vi "Configure Analysis.vi"(0 "VISA resource name":refnum<visa-resource-name>, 1 "Range Coupling (F:Disable)":bool, 2 "Peak Excursion (3.0)":dbl=3.0 format="%^.2e", 3 "Peak Polarity (0: Positive)":u16(ring) items=["Positive", "Negative", "Both"], 4 "Partial Range Analysis State (F:Disable)":bool, 5 "error in (no error)":errorcluster, 6 "Channel (1)":i32=1, 7 "Target Value (0.0)":dbl format="%^.2e", 8 "Analysis Type (0: Peak to Peak)":u16(ring) items=["Peak to Peak", "Standard Deviation", "Mean", "Maximum", "Minimum", "Peak", "All Peaks", "All Targets"], 9 "Target Polarity (0: Positive)":u16(ring) items=["Positive", "Negative", "Both"], 10 "Start (0.0)":dbl format="%^.2e", 11 "Stop (0.0)":dbl format="%^.2e") -> (14 "VISA resource name out":refnum<visa-resource-name>, 19 "error out":errorcluster)   [LabVIEW 2022 SP3, in "Agilent ENA Series.lvlib"]
doc: "Configures the analysis parameters.\n\n<b>Note:</b>\nThis VI is not supported by the E5080A and E5080B."
uses:
  <instrlib>/Agilent ENA Series/Agilent ENA Series.lvlib
panel:
  # "Note:\nThis VI is not supported by the E5080A and E5080B."
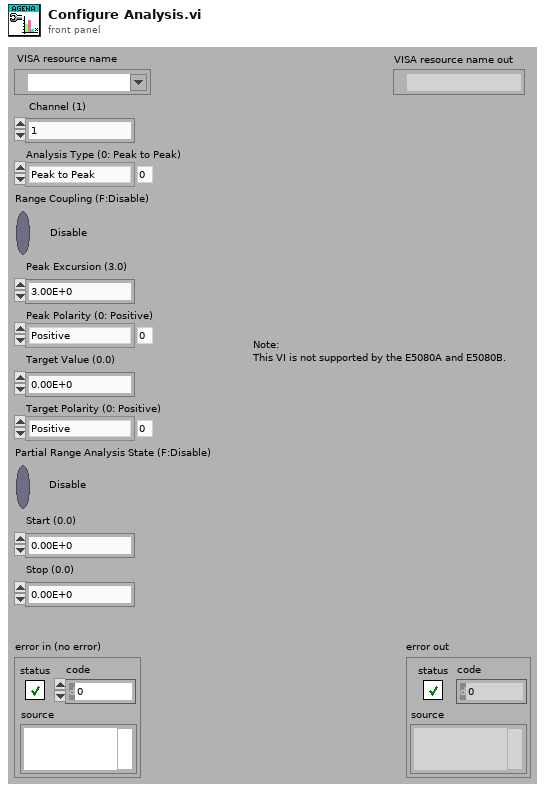
[diagram p1: front panel]
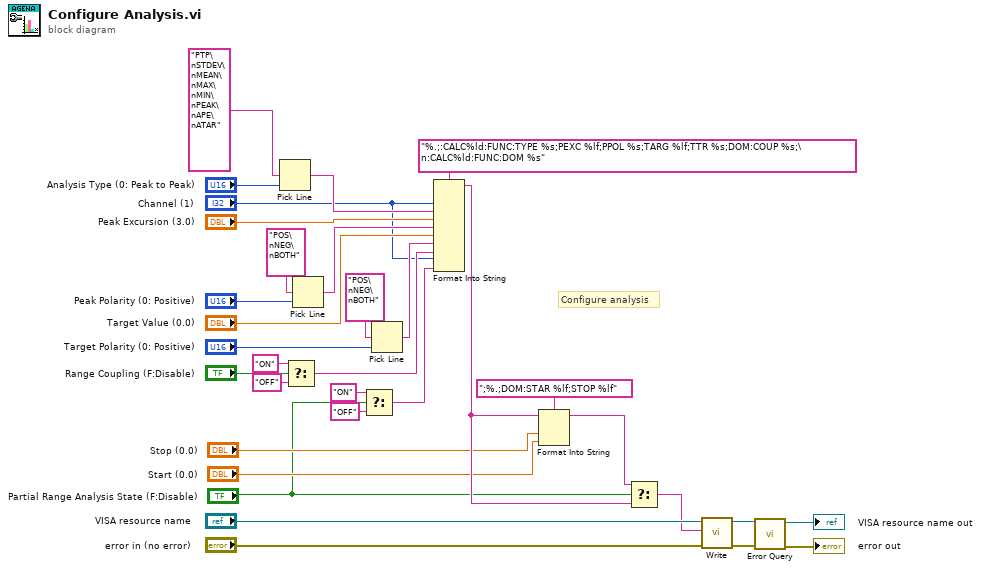
[diagram p0: block diagram]
diagram:
  # "Configure analysis"
  n1 = Pick Line(multi-line string="PTP\nSTDEV\nMEAN\nMAX\nMIN\nPEAK\nAPE\nATAR", line index="Analysis Type (0: Peak to Peak)") -> (output string=w25:string)  [unwired: 1 in]
  n2 = Select(t="ON", s="Range Coupling (F:Disable)", f="OFF") -> (s? t:f=w16:string)
  n3 = Pick Line(multi-line string="POS\nNEG\nBOTH", line index="Peak Polarity (0: Positive)") -> (output string=w21:string)  [unwired: 1 in]
  n4 = Select(t="ON", s="Partial Range Analysis State (F:Disable)", f="OFF") -> (s? t:f=w2:string)
  n5 = Pick Line(multi-line string="POS\nNEG\nBOTH", line index="Target Polarity (0: Positive)") -> (output string=w17:string)  [unwired: 1 in]
  n6 = Format Into String(format string="%.;:CALC%ld:FUNC:TYPE %s;PEXC %lf;PPOL %s;TARG %lf;TTR %s;DOM:COUP %s;\n:CALC%ld:FUNC:DOM %s", "Channel (1)", w25, "Peak Excursion (3.0)", w21, "Target Value (0.0)", w17, w16, "Channel (1)", w2) -> (resulting string=w10:string)  [unwired: 2 in, 1 out]
  n7 = Format Into String(format string=";%.;DOM:STAR %lf;STOP %lf", initial string=w10, "Stop (0.0)", "Start (0.0)") -> (resulting string=w9:string)  [unwired: 1 in, 1 out]
  n8 = Select(t=w9, s="Partial Range Analysis State (F:Disable)", f=w10) -> (s? t:f=w6:string)
  n9 = call <instrlib>:"Write.vi"("error in (no error)"="error in (no error)", "String ()"=w6, "VISA resource name"="VISA resource name") -> ("error out"=w14:errorcluster, "VISA resource name out"=w15:refnum<visa-resource-name>)  [unwired: 6 in, 1 out]
  n10 = call <instrlib>:"Error Query.vi"("error in (no error)"=w14, "VISA resource name"=w15) -> ("error out"=→"error out":errorcluster, "VISA resource name out"=→"VISA resource name out":refnum<visa-resource-name>)  [unwired: 6 in, 2 out]
